vi "Main.vi"() -> ()   [LabVIEW 2014]
panel:
  out "Progress":i32(slide) scale=0.0..3.0
  in  "Start building":bool
  in  "Select piece":i32
  in  "Down":bool
  in  "Right":bool
  in  "Left":bool
  in  "Up":bool
  in  "stop":bool
  in  "Place piece":bool
  in  "Select piece type":i32
  out "2D Picture":picture
  # "Wait a minute"
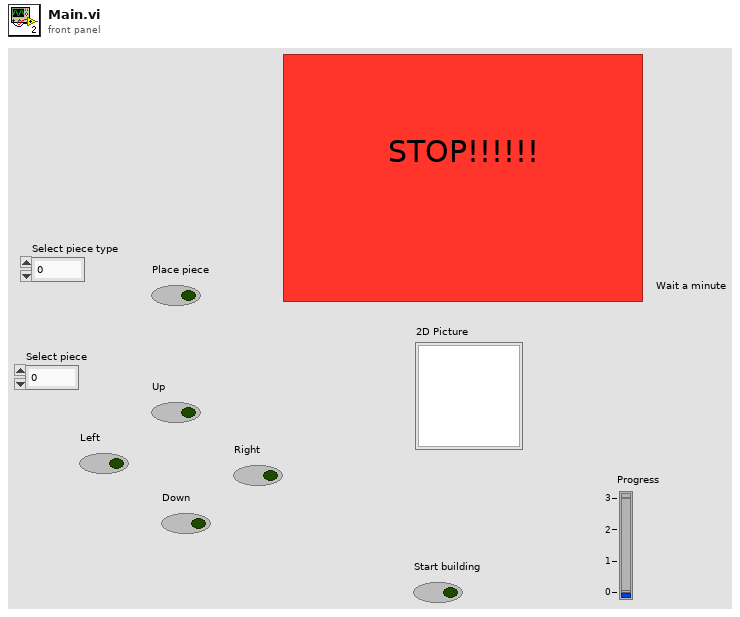
[diagram p1: front panel]
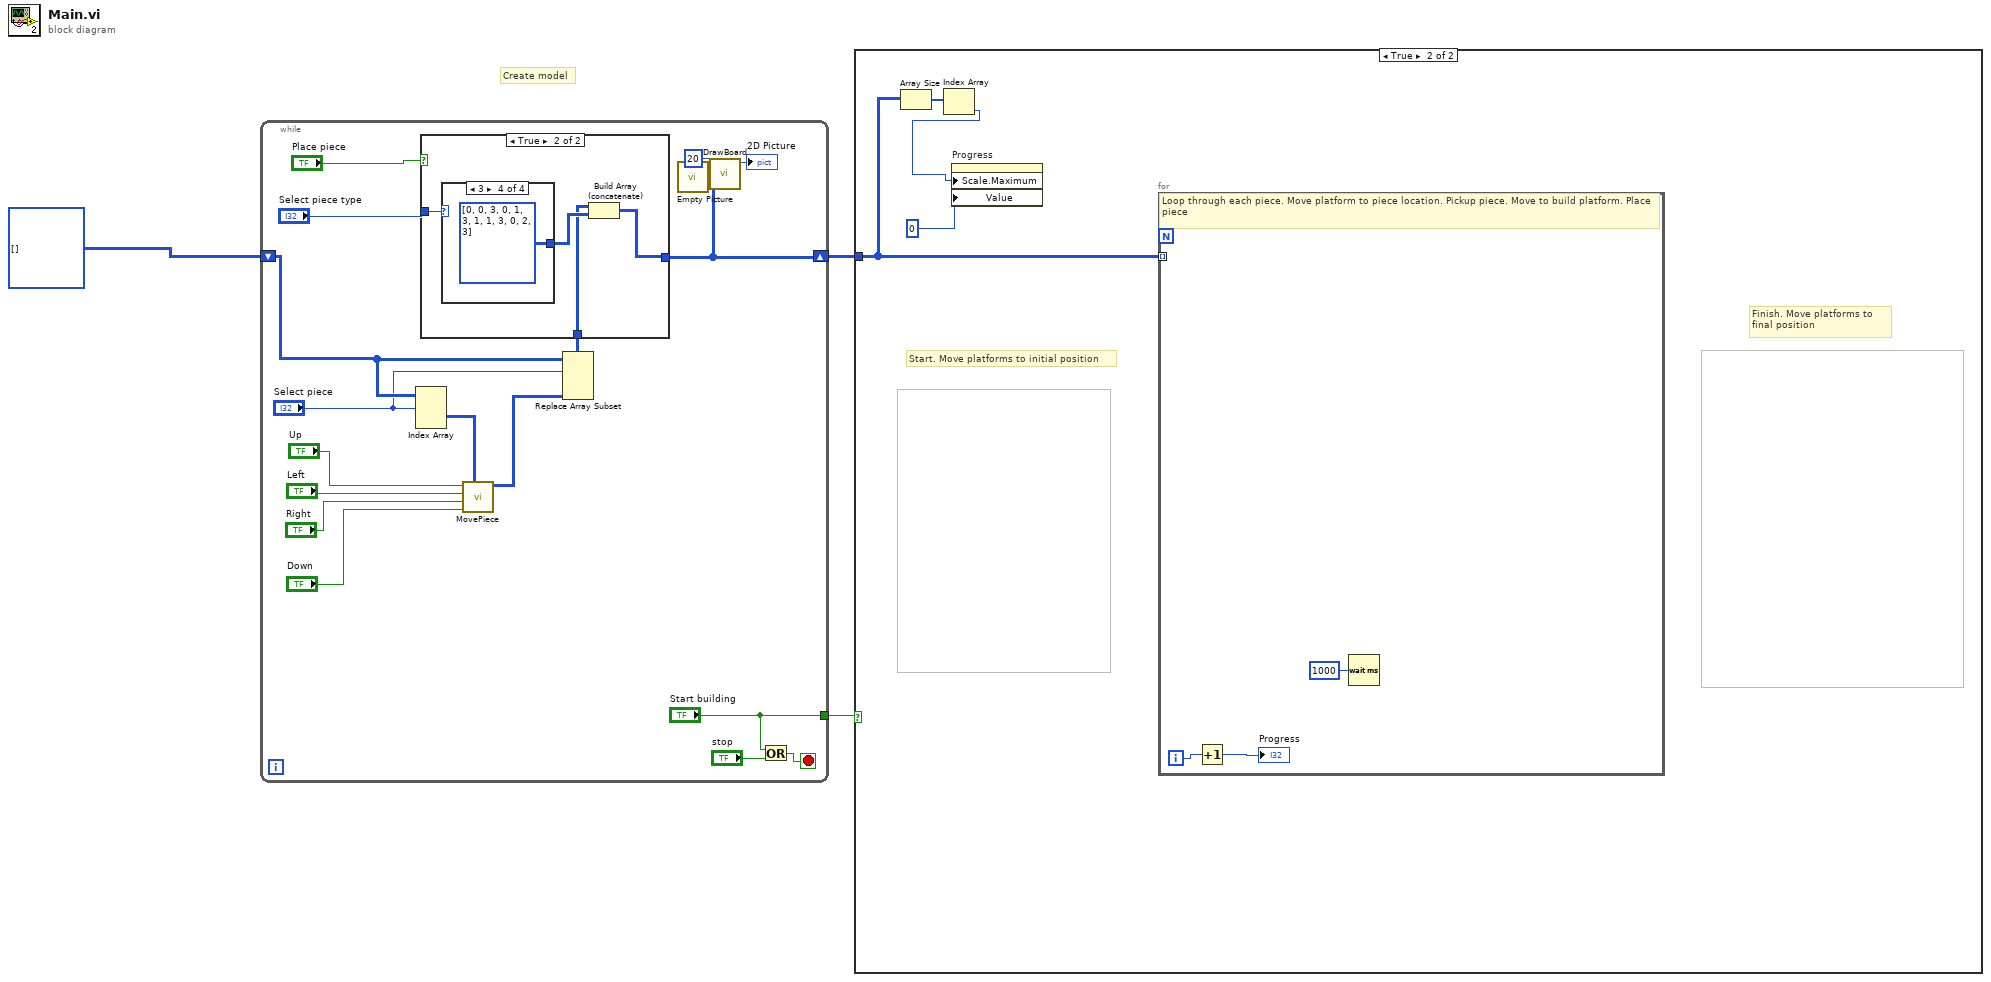
[diagram p0: block diagram]
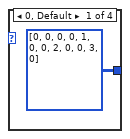
[diagram p4: hidden frame]
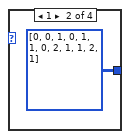
[diagram p5: hidden frame]
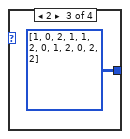
[diagram p6: hidden frame]
diagram:
  # "Create model"
  n1 = while {
    shift-right: [w14] -> w1
    shift-left: i32[][][] [] -> [w19]
    tunnel: ["Start building"] -> w2
    stop <- w6 stop-if-true
    n2 = Index Array(array=w19, index (dim 0)="Select piece") -> (element=w7:i32[][])  [unwired: 2 in]
    n3 = call "MovePiece.vi"("Old piece"=w7, "Down"="Down", "Right"="Right", "Left"="Left", "Up"="Up") -> ("New piece"=w17:i32[][])  [unwired: 6 in]
    n4 = Replace Array Subset(array=w19, new element=w17, index (dim 0)="Select piece") -> (w16:i32[][][])  [unwired: 2 in]
    n5 = case shown="True" "Place piece" {
      tunnel: "Select piece type" -> [_ w26]
      tunnel: [w22 w24] -> w14
      tunnel: w16 -> [w22 w23]
      frame False {
      }
      frame True {
        n6 = case shown="3" w26 {
          tunnel: [i32[][] [[0, 0, 0], [0, 1, 0], [0, 2, 0], [0, 3, 0]] i32[][] [[0, 0, 1], [0, 1, 1], [0, 2, 1], [1, 2, 1]] i32[][] [[1, 0, 2], [1, 1, 2], [0, 1, 2], [0, 2, 2]] i32[][] [[0, 0, 3], [0, 1, 3], [1, 1, 3], [0, 2, 3]]] -> w25
          frame 0, Default {
          }
          frame 1 {
          }
          frame 2 {
          }
          frame 3 {
          }
        }
        n7 = Build Array (concatenate)(w23, w25) -> (w24:i32[][][])
      }
    }
    n8 = call "Empty Picture"() -> ("empty picture"=w15:picture)
    n9 = call "DrawBoard.vi"("picture in"=w15, "Pieces"=w14, "Block Size"=i16 20) -> ("picture out"=→"2D Picture":picture)  [unwired: 8 in]
    n10 = Or(x="Start building", y="stop") -> (x .or. y?=w6:bool)
  }
  n11 = case shown="True" w2 {
    tunnel: w1 -> [_ w34]
    frame False {
    }
    frame True {
      # "Finish. Move platforms to \nfinal position"
      # "Start. Move platforms to initial position"
      n12 = Array Size(array=w34) -> (size(s)=w33:i32[])
      n13 = Index Array(array=w33) -> (element=w31:i32)  [unwired: 1 in]
      n14 = property on="Progress" class="Slide (strict)"("Scale.Maximum"=w31, "Value"=0 ("Progress")) -> ()  [unwired: 2 in, 2 out]
      n15 = for {
        tunnel: w34 -> [_] mode=indexing
        i -> [w37]
        # "Loop through each piece. Move platform to piece location. Pickup piece. Move to build platform. Place piece"
        n16 = Increment(x=w37) -> (x+1=→"Progress":i32)
        n17 = Wait (ms)(milliseconds to wait=u32 1000) -> ()  [unwired: 1 out]
      }
    }
  }
